vi "CreateError.vi"(11 "error":errorcluster) -> (3 "EventData":refnum<class "EventData.lvclass">)   [LabVIEW 2016, in "Event Logging.lvlib" / "EventData.lvclass"]
uses:
  EventData.lvclass
  Types/EventType.ctl
  EventData.lvclass/EventData.ctl
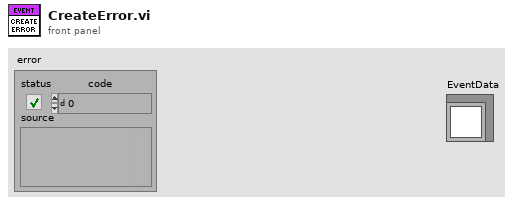
[diagram p1: front panel]
types:
  T1 = typedef "Event Logging.lvlib/EventData.lvclass/EventType.ctl" = enum16{"Event", "Warning", "Error"}
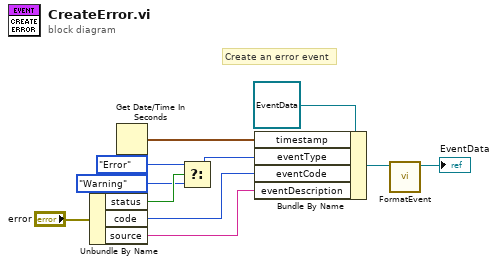
[diagram p0: block diagram]
diagram:
  # "Create an error event"
  n1 = Unbundle By Name("error") -> ("status"=w6:bool, "code"=w2:i32, "source"=w1:string)
  n2 = Get Date/Time In Seconds() -> (seconds since 1Jan1904=w10:timestamp)
  n3 = Select(t=EventType."Error" ("eventType"), s=w6, f=EventType."Warning" ("eventType")) -> (s? t:f=w3:T1)
  n4 = Bundle By Name(cluster=refnum<class "EventData.lvclass"> refnum ("Event Logging.lvlib:EventData.lvclass"), "timestamp"=w10, "eventType"=w3, "eventCode"=w2, "eventDescription"=w1) -> (w9:refnum<class "EventData.lvclass">)
  n5 = call-dynamic "FormatEvent.vi"("EventData in"=w9) -> ("EventData out"=→"EventData":refnum<class "EventData.lvclass">)  [unwired: 10 in]
